vi "Write Compass Data.vi"(8 "error in (no error)":errorcluster, 10 "Compass Data":T1, 11 "Compass Data Message in":refnum<class "Compass Data Message.lvclass">) -> (0 "error out":errorcluster, 3 "Compass Data Message out":refnum<class "Compass Data Message.lvclass">)   [LabVIEW 2015, in "RDS Child Messages.lvlib" / "Compass Data Message.lvclass"]
uses:
  Compass Data Message.lvclass
  RDS Instruments/Compass/Compass Data.ctl
  Compass Data Message.lvclass/Compass Data Message.ctl
  RDS Instruments/RDS Instrument Library.lvlib
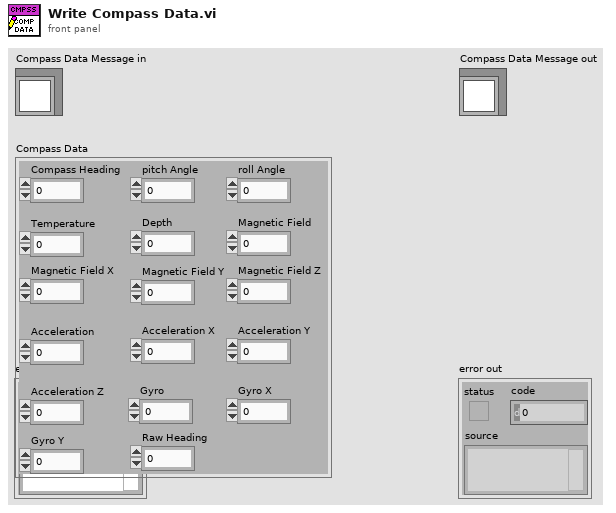
[diagram p1: front panel]
types:
  T1 = typedef "RDS Instrument Library.lvlib/Compass Data.ctl" = cluster{"Compass Heading":sgl, "pitch Angle":sgl, "roll Angle":sgl, "Temperature":sgl, "Depth":sgl, "Magnetic Field":sgl, "Magnetic Field X":sgl, "Magnetic Field Y":sgl, "Magnetic Field Z":sgl, "Acceleration":sgl, "Acceleration X":sgl, "Acceleration Y":sgl, "Gyro":sgl, "Gyro X":sgl, "Acceleration Z":sgl, "Gyro Y":sgl, "Raw Heading":sgl}
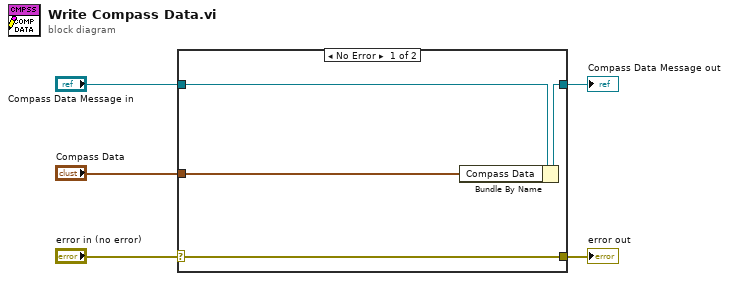
[diagram p0: block diagram]
diagram:
  n1 = case shown="No Error" "error in (no error)" {
    selector: "error in (no error)" -> [w9 w10]
    tunnel: [w9 w10] -> w4
    tunnel: [w7 w11] -> w2
    tunnel: "Compass Data Message in" -> [w8 w11]
    tunnel: "Compass Data" -> [w6 _]
    frame No Error {
      n2 = Bundle By Name(cluster=w8, "Compass Data"=w6) -> (w7:refnum<class "Compass Data Message.lvclass">)
    }
    frame Error {
    }
  }
  "error out" <- w4
  "Compass Data Message out" <- w2
